vi "NI-DCPower Source DC Voltage.vi"() -> ()   [LabVIEW 2021]
doc: "Demonstrates how to use the DC Voltage Output Function to force an output voltage. This example initializes a session, configures the Output Function, Sense, Autorange, Voltage Level and Current Limit, initiates generation, waits for a specified delay, and measures the voltage and current output. This example uses Single Point source mode."
uses:
  <instrlib>/niDCPower/nidcpower.llb/niDCPower Source Mode.ctl
  <instrlib>/niDCPower/nidcpower.llb/niDCPower Wait For Event - Event.ctl
  <instrlib>/niDCPower/nidcpower.llb/niDCPower Output Function.ctl
  <instrlib>/niScope/Acquire/niScope Multi Read Cluster.vi
panel:
  in  "Scope Channel(s)":string="0" caption="Channel(s)"
  in  "Scope":refnum<k15>="Dev1" caption="Resource Name(s)"
  out "Waveform Graph":T1(graph)
  in  "error in":errorcluster
  out "error out":errorcluster
  in  "Source Delay (Sec)":dbl=0.1 format="%.3p"
  out "Voltage Measurement":dbl
  out "Current Measurement":dbl
  in  "Current Limit Range":dbl=0.01 format="%.3p"
  in  "Voltage Level Range":dbl=6.0 format="%.5p"
  in  "Current Limit":dbl=0.01 format="%.3p"
  in  "Voltage Level":dbl=2.0 format="%.5p"
  in  "Vin SMU Channel":string="0"
  in  "Vin SMU":refnum<k15>="Dev1"
  # "Overview: Demonstrates how to use the DC Voltage Output Function to force an output voltage.  \nThis example initializes a session; configures the Output Function, Voltage Level and Current Limit; \ninitiates generation; waits for a specified delay; and measures the voltage and current output. \nRequirements: NI-DCPower\nInstructions:\n1. Select the appropriate device in the Resource Name control.\n2. Configure the parameters of the DC Voltage signal you'd like to output.\n3. Run the VI."
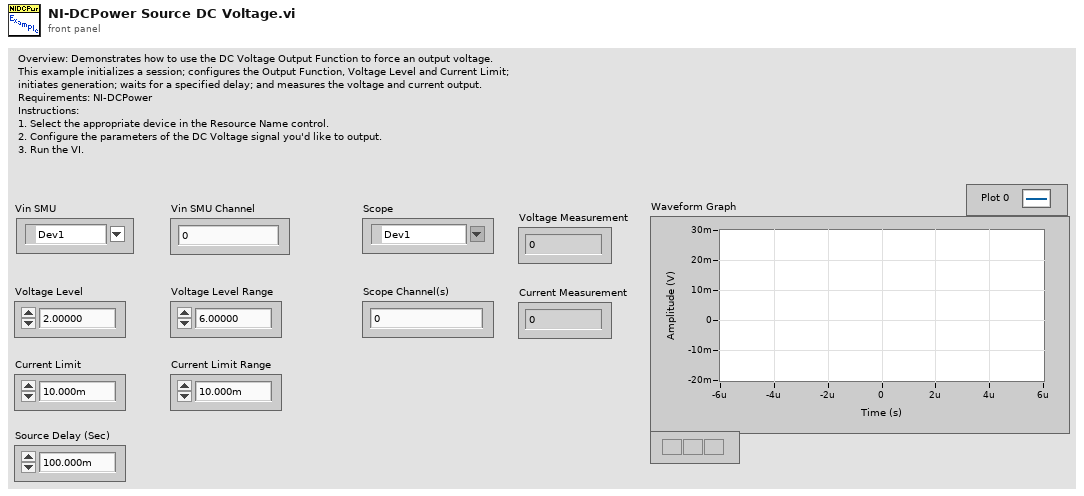
[diagram p1: front panel]
types:
  T1 = cluster{"relativeInitialX":dbl, "xIncrement":dbl, "wfm":dbl[]}[]
  T2 = typedef "niDCPower Output Function.ctl" = i32
  T3 = typedef "niDCPower Wait For Event - Event.ctl" = i32
  T4 = typedef "niDCPower Source Mode.ctl" = i32
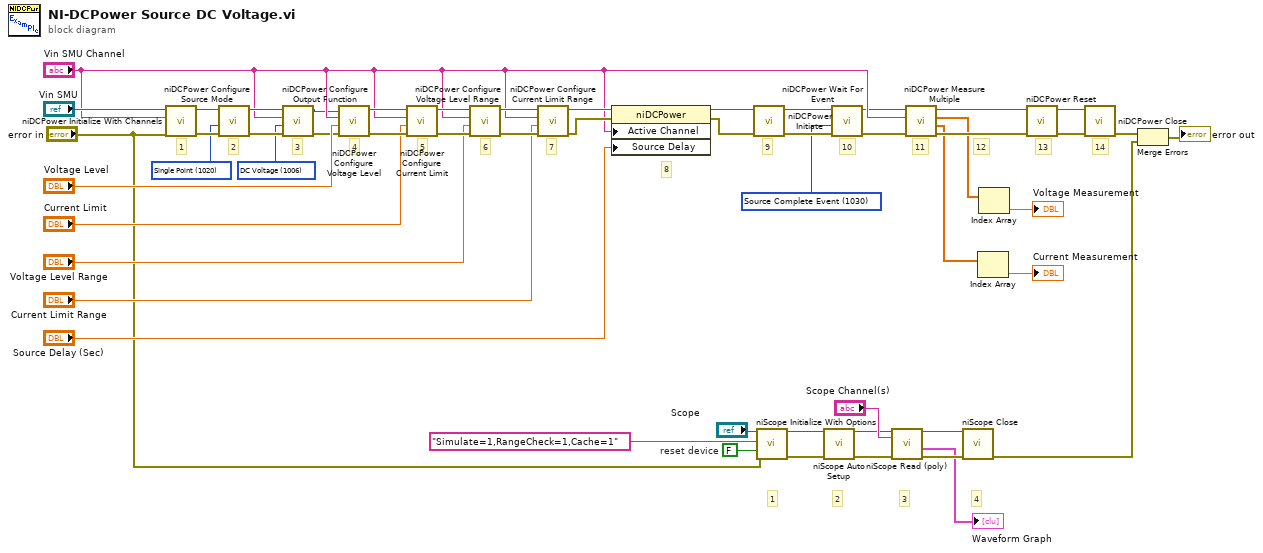
[diagram p0: block diagram]
diagram:
  w7 = FALSE  # reset device
  w20 = T2 1006 items=["DC Voltage"=1006, "DC Current"=1007, "Pulse Voltage"=1049, "Pulse Current"=1050] ("output function")
  w23 = T3 1030 items=["Source Complete Event"=1030, "Measure Complete Event"=1031, "Sequence Iteration Complete Event"=1032, "Sequence Engine Done Event"=1033] ("event")
  w42 = T4 1020 items=["Single Point"=1020, "Sequence"=1021] ("source mode")
  # "4"
  # "3"
  # "2"
  # "1"
  # "14"
  # "9"
  # "11"
  # "10"
  # "7"
  # "6"
  # "2"
  # "3"
  # "12"
  # "13"
  # "8"
  # "5"
  # "4"
  # "1"
  n1 = call <instrlib>:"niDCPower Initialize With Channels.vi"("error in (no error)"="error in", "channels"="Vin SMU Channel", "resource name"="Vin SMU") -> ("error out"=w46:errorcluster, "instrument handle out"=w45:refnum<k15>)  [unwired: 2 in, 5 out]
  n2 = call <instrlib>:"niDCPower Configure Source Mode.vi"("error in (no error)"=w46, "source mode"=w42, "instrument handle"=w45) -> ("error out"=w44:errorcluster, "instrument handle out"=w43:refnum<k15>)  [unwired: 7 out]
  n3 = call <instrlib>:"niDCPower Configure Output Function.vi"("error in (no error)"=w44, "output function"=w20, "channel name"="Vin SMU Channel", "instrument handle"=w43) -> ("error out"=w21:errorcluster, "instrument handle out"=w22:refnum<k15>)  [unwired: 6 out]
  n4 = call <instrlib>:"niDCPower Configure Voltage Level.vi"("error in (no error)"=w21, "voltage level"="Voltage Level", "channel name"="Vin SMU Channel", "instrument handle"=w22) -> ("error out"=w51:errorcluster, "instrument handle out"=w52:refnum<k15>)  [unwired: 6 out]
  n5 = call <instrlib>:"niDCPower Configure Current Limit.vi"("error in (no error)"=w51, "current limit"="Current Limit", "channel name"="Vin SMU Channel", "instrument handle"=w52) -> ("error out"=w41:errorcluster, "instrument handle out"=w40:refnum<k15>)  [unwired: 1 in, 5 out]
  n6 = call <instrlib>:"niDCPower Configure Voltage Level Range.vi"("error in (no error)"=w41, "voltage level range"="Voltage Level Range", "channel name"="Vin SMU Channel", "instrument handle"=w40) -> ("error out"=w39:errorcluster, "instrument handle out"=w38:refnum<k15>)  [unwired: 6 out]
  n7 = call <instrlib>:"niDCPower Configure Current Limit Range.vi"("error in (no error)"=w39, "current limit range"="Current Limit Range", "channel name"="Vin SMU Channel", "instrument handle"=w38) -> ("error out"=w30:errorcluster, "instrument handle out"=w33:refnum<k15>)  [unwired: 6 out]
  n8 = property class="niDCPower"(reference=w33, error in=w30, "Active Channel"="Vin SMU Channel", "Source Delay"="Source Delay (Sec)") -> (reference out=w32:refnum<k15>, error out=w31:errorcluster)
  n9 = call <instrlib>:"niDCPower Initiate.vi"("error in (no error)"=w31, "instrument handle"=w32) -> ("error out"=w25:errorcluster, "instrument handle out"=w27:refnum<k15>)  [unwired: 2 in, 6 out]
  n10 = call <instrlib>:"niScope Initialize With Options.vi"("resource name"="Scope", "option string"="Simulate=1,RangeCheck=1,Cache=1", "reset device"=w7, "error in"="error in") -> ("instrument handle"=w4:refnum<k15>, "error out"=w5:errorcluster)  [unwired: 10 in]
  n11 = call <instrlib>:"niScope Auto Setup.vi"("instrument handle"=w4, "error in"=w5) -> ("instrument handle out"=w8:refnum<k15>, "error out"=w9:errorcluster)  [unwired: 12 in]
  n12 = call <instrlib>:"niDCPower Wait For Event.vi"("error in (no error)"=w25, "event"=w23, "instrument handle"=w27) -> ("error out"=w24:errorcluster, "instrument handle out"=w26:refnum<k15>)  [unwired: 1 in, 6 out]
  n13 = call-poly <instrlib>:"niScope Read (poly).vi"("error in"=w9, "channels"="Scope Channel(s)", "instrument handle"=w8) -> ("error out"=w12:errorcluster, "waveform"=→"Waveform Graph":T1, "instrument handle out"=w13:refnum<k15>)  [unwired: 5 in, 1 out]
  n14 = call <instrlib>:"niDCPower Measure Multiple.vi"("error in (no error)"=w24, "channel name"="Vin SMU Channel", "instrument handle"=w26) -> ("error out"=w34:errorcluster, "current measurements"=w18:dbl[], "voltage measurements"=w16:dbl[], "instrument handle out"=w35:refnum<k15>)  [unwired: 5 out]
  n15 = call <instrlib>:"niScope Close.vi"("instrument handle"=w13, "error in"=w12) -> ("error out"=w2:errorcluster)  [unwired: 13 in]
  n16 = Index Array(array=w18) -> (element=→"Current Measurement":dbl)  [unwired: 1 in]
  n17 = Index Array(array=w16) -> (element=→"Voltage Measurement":dbl)  [unwired: 1 in]
  n18 = call <instrlib>:"niDCPower Reset.vi"("error in (no error)"=w34, "instrument handle"=w35) -> ("error out"=w48:errorcluster, "instrument handle out"=w49:refnum<k15>)  [unwired: 2 in, 6 out]
  n19 = call <instrlib>:"niDCPower Close.vi"("error in (no error)"=w48, "instrument handle"=w49) -> ("error out"=w19:errorcluster)  [unwired: 9 out]
  n20 = Merge Errors(w19, w2) -> (→"error out":errorcluster)
